vi "raisePlatforms_2parts.vi"() -> ()   [LabVIEW 2017]
panel:
  in  "Platforms going...":string(combo)="up"
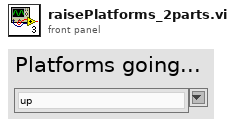
[diagram p1: front panel]
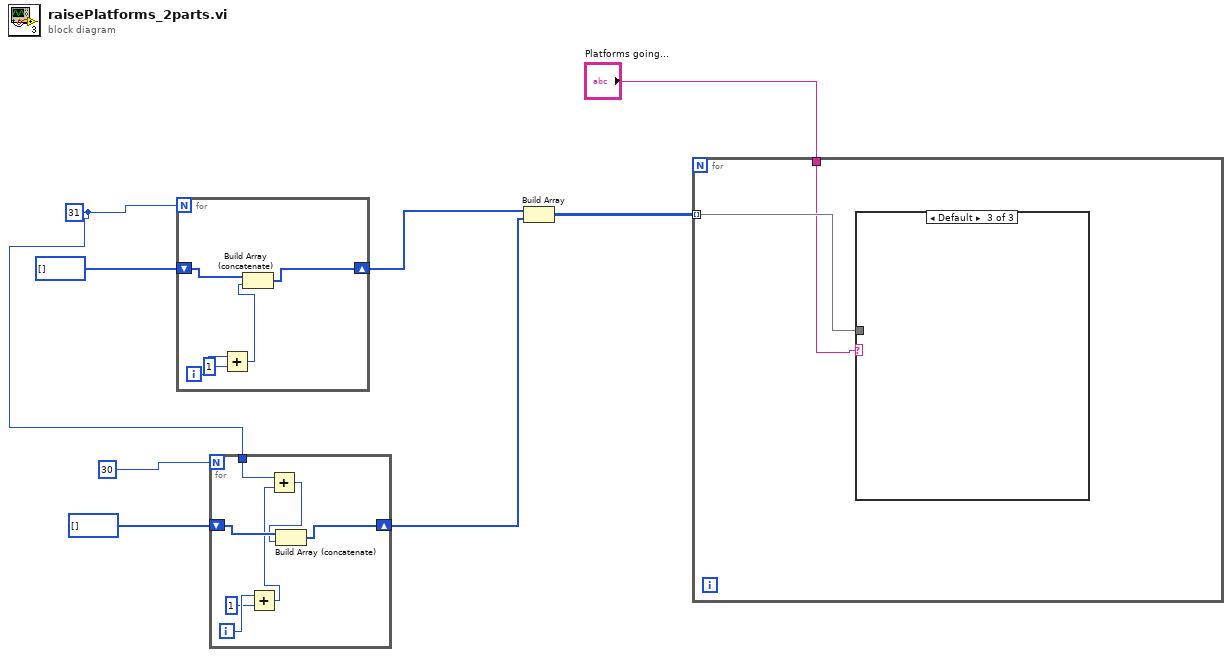
[diagram p0: block diagram]
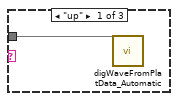
[diagram p2: hidden frame]
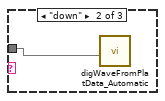
[diagram p3: hidden frame]
diagram:
  w3 = 31 ("Numeric")
  n1 = for {
    N: w3 -> [_]
    shift-right: [w12] -> w6
    shift-left: i32[] [] -> [w13]
    i -> [w11]
    n2 = Add(x=w11, y=1) -> (x+y=w9:i32)
    n3 = Build Array (concatenate)(w13, w9) -> (w12:i32[])
  }
  n4 = for {
    N: 30 ("Numeric") -> [_]
    shift-right: [w19] -> w2
    shift-left: i32[] [] -> [w20]
    tunnel: w3 -> [w18]
    i -> [w16]
    n5 = Add(x=w16, y=1) -> (x+y=w14:i32)
    n6 = Add(x=w18, y=w14) -> (x+y=w17:i32)
    n7 = Build Array (concatenate)(w20, w17) -> (w19:i32[])
  }
  n8 = Build Array(w6, w2) -> (w8:i32[][])
  n9 = for {
    tunnel: w8 -> [w22] mode=indexing
    tunnel: "Platforms going..." -> [w21]
    n10 = case shown="Default" w21 {
      tunnel: w22 -> [w23 w24 _]
      frame "up" {
        n11 = call "digWaveFromPlatData_Automatic.vi"("Platforms\nto raise"=w23) -> ()  [unwired: 10 in, 1 out]
      }
      frame "down" {
        n12 = call "digWaveFromPlatData_Automatic.vi"("Platforms\nto lower"=w24) -> ()  [unwired: 10 in, 1 out]
      }
      frame Default {
      }
    }
  }
